vi "FPGAkeeprunning.vi"() -> ()   [LabVIEW 2019]
uses:
  RSNRPZ/RSNRPZcontrol.ctl
  <vilib>/FPGAPlugInAG/PXI-7842R/niLvFpga_Open_PXI-7842R.vi
  <vilib>/rvi/interface/common/dynamic/niFpgaDynamicAddResources.vi
  <vilib>/Utility/error.llb/Error Cluster From Error Code.vi
  <vilib>/rvi/errors/niLvFpgaAdjustHostInterfaceError.vi
  <vilib>/rvi/interface/common/niFpgaWaitOnOcc.vi
  <instrlib>/Agilent 3446X Series/Public/Data/Read (Single Point).vi
  <vilib>/FPGAPlugInAG/Dynamic/niLvFpga_Close_Dynamic.vi
  <vilib>/rvi/interface/nirviOpenFPGA/nirviOpenFPGA.xnode
  FPGA_bitfile/Jarvis_FPGATargetMacro_281119TDCLV2017_HUsPPJBlkv4.lvbitx
  <vilib>/rvi/interface/nirviReadWriteControl/nirviReadWriteControl.xnode
  <vilib>/rvi/interface/nirviMethod/nirviMethod.xnode
  <vilib>/rvi/interface/nirviCloseFPGA/nirviCloseFPGA.xnode
  NiFpgaLv.dll
  <vilib>/rvi/interface/Simulation/niFpgaSimulationCallBeginRW.vi
  <vilib>/FPGAPlugInAG/Dynamic/niLvFpga_ConfigureFifo_Dynamic.vi
  <vilib>/rvi/errors/niLvFpgaMergeErrorWithErrorCode.vi
  <instrlib>/Agilent 3446X Series/Agilent 3446X Series.lvlib
panel:
  in  "file (use dialog)":path
  in  "stop":bool
  in  "RSNPRZsettings":T1={"Average Counts :"=1.0, "Correction Freq [MHz] :"=50.0, "Integration Time [ms] : "=0.1, "P :"=0.0, "I :"=0.0, "D :"=0.0, "Power setpoint :"=0.0, "PID on :"=FALSE, "Voltage :"=0.0, "Reset :"=FALSE, "Agilient Power Level [dBm] :"=0.0} caption="RSNPRZ Settings :" {"Agilient Power Level [dBm] :" format="%_3g"; "Voltage :" format="%_5g"; "Power setpoint :" format="%_4g"; "D :" format="%_4g"; "I :" format="%_4g"; "P :" format="%_4g"; "Integration Time [ms] :" format="%_3g"; "Correction Freq [MHz] :" format="%_4g"}
  out "FPGAerr":bool=TRUE
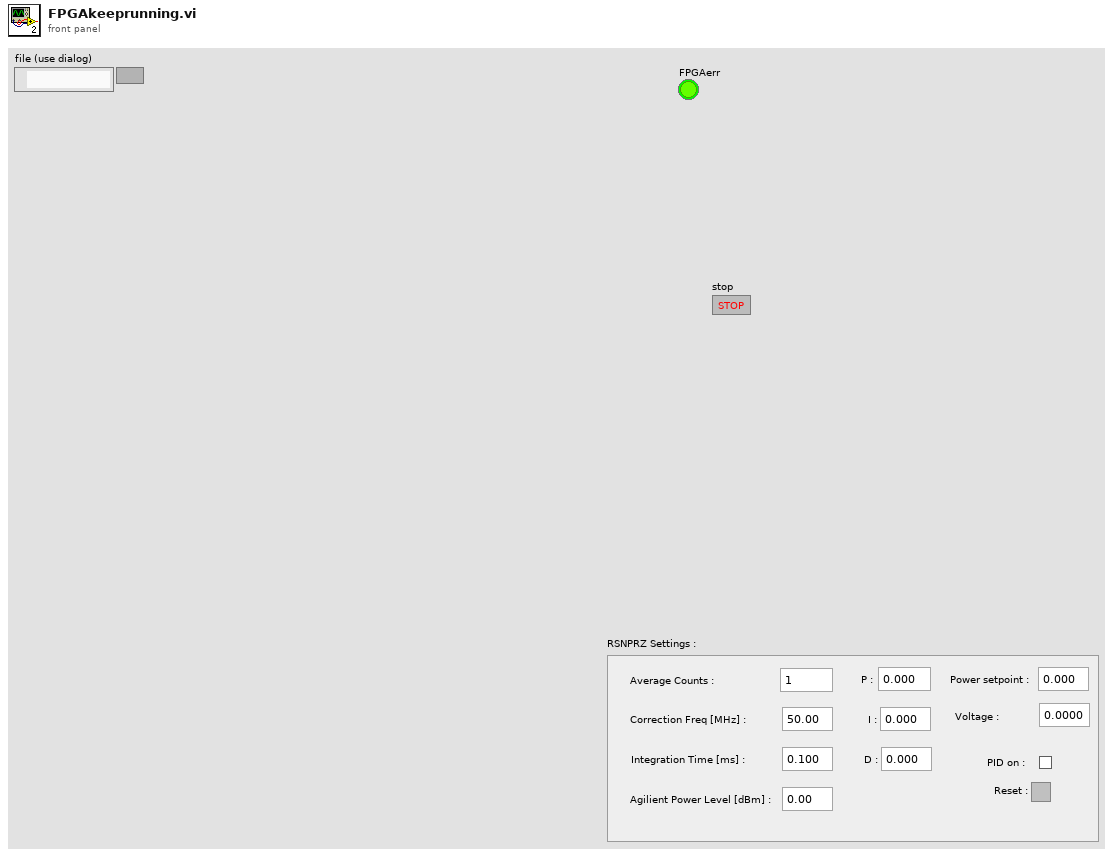
[diagram p1: front panel]
types:
  T1 = typedef "RSNRPZcontrol.ctl" = cluster{"Average Counts :":dbl, "Correction Freq [MHz] :":dbl, "Integration Time [ms] : ":dbl, "P :":dbl, "I :":dbl, "D :":dbl, "Power setpoint :":dbl, "PID on :":bool, "Voltage :":dbl, "Reset :":bool, "Agilient Power Level [dBm] :":dbl}
  T2 = cluster{"HighPowerNum":dbl, "LowPowerNum":dbl, "PIDnum":dbl, "DeltaFreq":dbl, "BaseFreq":dbl, "AOMout":dbl, "ButtonSelected":enum16{"PID", "Low", "High"}, "AO3":bool}
  T3 = cluster{"DIO 0":bool, "DIO 1":bool, "DIO 2":bool, "DIO 3":bool, "DIO 4":bool, "DIO 5":bool, "DIO 6":bool, "DIO 7":bool, "DIO 8":bool, "DIO 9":bool, "DIO 10":bool, "DIO 11":bool, "DIO 12":bool, "DIO 13":bool, "DIO 14":bool, "DIO 15":bool, "DIO 16":bool, "DIO 17":bool, "DIO 18":bool, "DIO 19":bool, "DIO 20":bool, "DIO 21":bool, "DIO 22":bool, "DIO 23":bool, "DIO 24":bool, "DIO 25":bool, "DIO 26":bool, "DIO 27":bool, "DIO 28":bool, "DIO 29":bool, "DIO 30":bool, "DIO 31":bool, "DIO 32":bool, "DIO 33":bool, "DIO 34":bool, "DIO 35":bool, "DIO 36":bool, "DIO 37":bool, "DIO 38":bool, "DIO 39":bool}
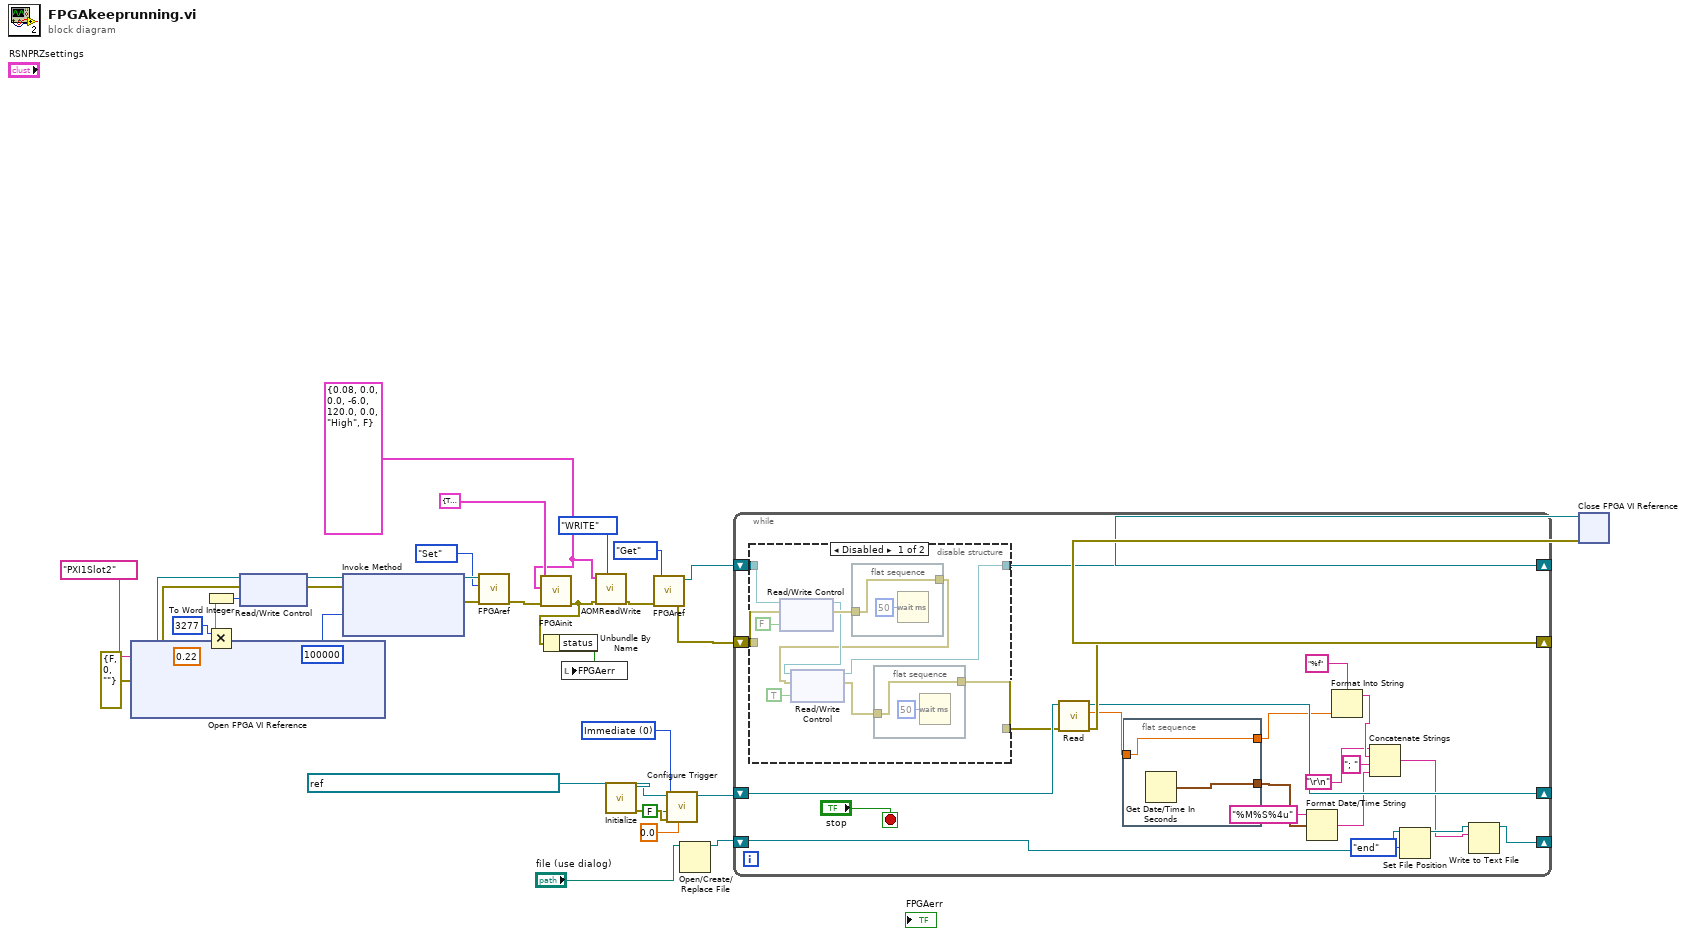
[diagram p0: block diagram]
diagram:
  w6 = 0 items=["Immediate", "Software (Bus)", "External", "Internal"] ("Trigger Source (0: Immediate)")
  w12 = T2 {"HighPowerNum"=0.08, "LowPowerNum"=0.0, "PIDnum"=0.0, "DeltaFreq"=-6.0, "BaseFreq"=120.0, "AOMout"=0.0, "ButtonSelected"=enum."High", "AO3"=FALSE} ("AOMsetting")
  n1 = xnode "Open FPGA VI Reference"("error in"=errorcluster {"status"=FALSE, "code"=0, "source"=""}, "resource name"=tag "PXI1Slot2") -> ("FPGA VI Reference Out"=w28:refnum<k20>, "error out"=w26:errorcluster)
  n2 = Multiply(x=3277, y=0.22) -> (x*y=w22:dbl)
  n3 = To Word Integer(number=w22) -> (16bit integer=w21:i16)
  n4 = xnode "Read/Write Control"("FPGA VI Reference In"=w28, "error in"=w26, "AO4 max"=w21) -> ("FPGA VI Reference Out"=w27:refnum<k20>, "error out"=w25:errorcluster)
  n5 = xnode "Invoke Method"("FPGA VI Reference In"=w27, "error in"=w25, "Requested Depth"=u32 100000) -> ("FPGA VI Reference Out"=w33:refnum<k20>, "error out"=w34:errorcluster)  [unwired: 1 out]
  n6 = call "FPGAref.vi"("error in"=w34, "Enum"=enum16{"Set", "Get"}."Set", "FPGA VI Reference Out"=w33) -> ("error out"=w31:errorcluster)  [unwired: 3 in, 1 out]
  n7 = call "FPGAinit.vi"("error in"=w31, "XAOMsetting"=w12, "DIOcluster"=T3 {"DIO 0"=TRUE, "DIO 1"=FALSE, "DIO 2"=FALSE, "DIO 3"=FALSE, "DIO 4"=FALSE, "DIO 5"=FALSE, "DIO 6"=FALSE, "DIO 7"=FALSE, "DIO 8"=FALSE, "DIO 9"=FALSE, "DIO 10"=FALSE, "DIO 11"=FALSE, "DIO 12"=TRUE, "DIO 13"=FALSE, "DIO 14"=FALSE, "DIO 15"=FALSE, "DIO 16"=FALSE, "DIO 17"=TRUE, "DIO 18"=FALSE, "DIO 19"=FALSE, "DIO 20"=FALSE, "DIO 21"=FALSE, "DIO 22"=FALSE, "DIO 23"=FALSE, "DIO 24"=FALSE, "DIO 25"=FALSE, "DIO 26"=FALSE, "DIO 27"=FALSE, "DIO 28"=FALSE, "DIO 29"=FALSE, "DIO 30"=FALSE, "DIO 31"=FALSE, "DIO 32"=FALSE, "DIO 33"=FALSE, "DIO 34"=FALSE, "DIO 35"=FALSE, "DIO 36"=FALSE, "DIO 37"=FALSE, "DIO 38"=FALSE, "DIO 39"=FALSE}) -> ("error out"=w19:errorcluster)  [unwired: 8 in]
  n8 = Unbundle By Name(w19) -> ("status"=w30:bool)
  n9 = local write "FPGAerr"(w30) -> ()
  n10 = call "AOMReadWrite.vi"("Enum"=enum16{"READ", "WRITE"}."WRITE", "error in"=w19, "XAOMsetting"=w12) -> ("error out"=w18:errorcluster)  [unwired: 6 in, 2 out]
  n11 = call <instrlib>:"Initialize.vi"("VISA resource name"=refnum<visa-resource-name> "USB0::0x2A8D::0x1401::MY53215765::INSTR") -> ("error out"=w7:errorcluster, "VISA resource name out"=w8:refnum<visa-resource-name>)  [unwired: 9 in]
  n12 = call "FPGAref.vi"("error in"=w18, "Enum"=enum16{"Set", "Get"}."Get") -> ("error out"=w14:errorcluster, "FPGA VI Reference Out 2"=w11:refnum<k20>)  [unwired: 4 in]
  n13 = call <instrlib>:"Configure Trigger.vi"("Manual Trigger Delay (1 s)"=0.0, "error in (no error)"=w7, "Auto Delay (T:Enable)"=FALSE, "Trigger Source (0: Immediate)"=w6, "VISA resource name"=w8) -> ("VISA resource name out"=w4:refnum<visa-resource-name>)  [unwired: 5 in, 1 out]
  n14 = Open/Create/Replace File(file path (use dialog)="file (use dialog)") -> (refnum out=w2:refnum<file>)  [unwired: 5 in, 2 out]
  n15 = while {
    shift-right: [w54] -> w10
    shift-left: w11 -> [w56]
    shift-right: [w51] -> w15
    shift-left: w14 -> [w55]
    shift-right: [w50] -> _
    shift-left: w4 -> [w53]
    shift-right: [w37] -> _
    shift-left: w2 -> [w41]
    stop <- "stop" stop-if-true
    n16 = disable-structure shown="Disabled" {
      disable-tunnel: w56 -> [w69 _]
      disable-tunnel: w55 -> [w63 _]
      disable-tunnel: [w61 _] -> w54
      disable-tunnel: [w60 _] -> w52
      frame Disabled {
        n17 = xnode "Read/Write Control"("FPGA VI Reference In"=w69, "error in"=w63, "D15"=FALSE) -> ("FPGA VI Reference Out"=w65:refnum<k20>, "error out"=w67:errorcluster)
        n18 = xnode "Read/Write Control"("FPGA VI Reference In"=w65, "error in"=w64, "D15"=TRUE) -> ("FPGA VI Reference Out"=w61:refnum<k20>, "error out"=w62:errorcluster)
        n19 = flat-sequence {
          tunnel: w67 -> [w72]
          tunnel: [w72] -> w64
          frame #0 {
            n20 = Wait (ms)(milliseconds to wait=u32 50) -> ()  [unwired: 1 out]
          }
        }
        n21 = flat-sequence {
          tunnel: w62 -> [w70]
          tunnel: [w70] -> w60
          frame #0 {
            n22 = Wait (ms)(milliseconds to wait=u32 50) -> ()  [unwired: 1 out]
          }
        }
      }
      frame Enabled {
      }
    }
    n23 = call-poly <instrlib>:"Read.vi"("error in (no error)"=w52, "VISA resource name"=w53) -> ("error out"=w51:errorcluster, "Measurement"=w49:dbl, "VISA resource name out"=w50:refnum<visa-resource-name>)  [unwired: 7 in]
    n24 = flat-sequence {
      tunnel: w49 -> [w58]
      tunnel: [w59] -> w44
      tunnel: [w58] -> w47
      frame #0 {
        n25 = Get Date/Time In Seconds() -> (seconds since 1Jan1904=w59:timestamp)
      }
    }
    n26 = Format Date/Time String(time format string (%c)="%M%S%4u", seconds (now)=w44) -> (date/time string=w43:string)  [unwired: 1 in]
    n27 = Format Into String(format string="%f", w47) -> (resulting string=w45:string)  [unwired: 2 in, 1 out]
    n28 = Concatenate Strings("\r\n", w45, "; " ("string"), w43) -> (w38:string)
    n29 = Set File Position(refnum=w41, from (0:start)=enum16{"start", "end", "current"}."end") -> (refnum out=w39:refnum<file>)  [unwired: 2 in, 1 out]
    n30 = Write to Text File(file (use dialog)=w39, text=w38) -> (refnum out=w37:refnum<file>)  [unwired: 2 in, 2 out]
  }
  n31 = xnode "Close FPGA VI Reference"("FPGA VI Reference In"=w10, "error in"=w15) -> ()  [unwired: 1 out]
